vi "INI-FGV2.vi"(6 "Enum":T1, 8 "Raw String? (F)":bool, 9 ">> Section >>":string, 10 ">> Default Value >>":string, 11 ">> Variable Name >>":string) -> (0 "error out":errorcluster, 2 "Key?":bool, 3 "Value":string)   [LabVIEW 2017, in "INI-Static-Variable-Support.lvlib"]
uses:
  INI-Static-Variable-Support.lvlib
  _fgv-oper.ctl
  global-csm-ini-db-change-flag.vi
  LabVIEW-Config/Read Key (String).vi
  LabVIEW-Config/LabVIEW-Config.lvlib
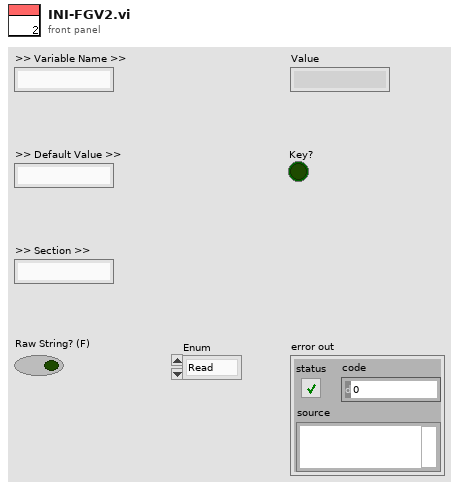
[diagram p1: front panel]
types:
  T1 = typedef "_fgv-oper.ctl" = enum16{"Read", "Write", "Sync"}
  T2 = typedef "LabVIEW-Config.lvlib/Config.ctl" = cluster{"Path":path, "Lines":string[], "Tokens":enum8{"comment", "section", "key"}[], "Modified?":bool}
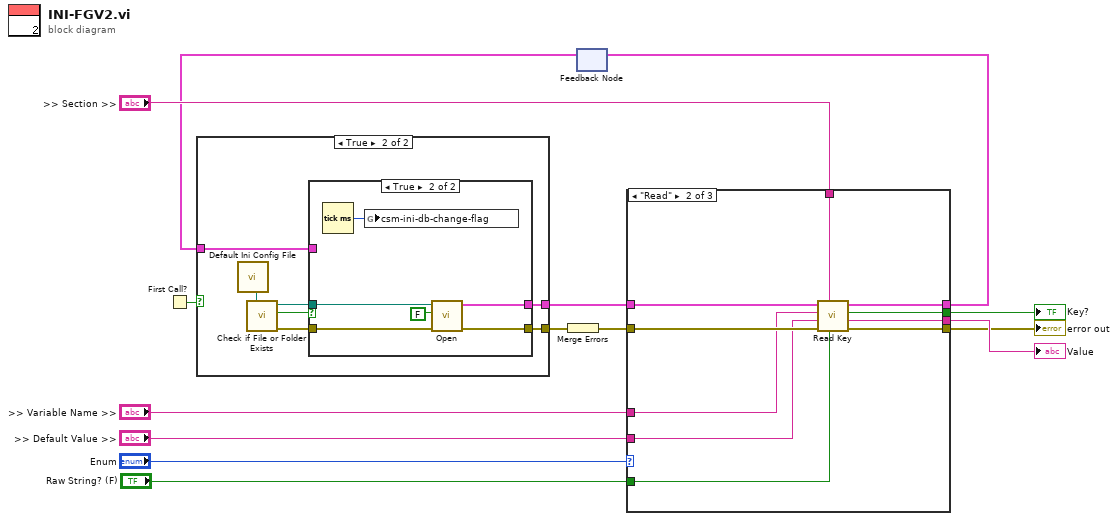
[diagram p0: block diagram]
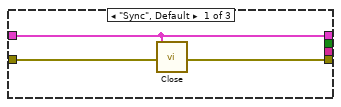
[diagram p2: hidden frame]
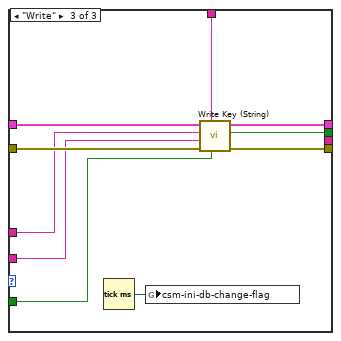
[diagram p3: hidden frame]
diagram:
  n1 = First Call?() -> (First Call?: T/F=w7:bool)
  n2 = feedback #1() -> (w4:T2)  [unwired: 1 in]
  n3 = case shown="True" w7 {
    tunnel: [w15 w19] -> w13
    tunnel: [_ w18] -> w6
    tunnel: w4 -> [w15 w16]
    frame False {
    }
    frame True {
      n4 = call "Default Ini Config File.vi"() -> ("appended path"=w22:path)  [unwired: 11 in]
      n5 = call <vilib>:"Check if File or Folder Exists.vi"("path"=w22) -> ("error out"=w20:errorcluster, "file or folder exists?"=w17:bool, "dup path"=w21:path)  [unwired: 8 in]
      n6 = case shown="True" w17 {
        tunnel: w21 -> [_ w30]
        tunnel: w20 -> [w24 w29]
        tunnel: [w23 w27] -> w19
        tunnel: [w24 w26] -> w18
        tunnel: w16 -> [w23 _]
        frame False {
        }
        frame True {
          n7 = Tick Count (ms)() -> (millisecond timer value=w25:u32)
          n8 = global write "global-csm-ini-db-change-flag.vi" "csm-ini-db-change-flag"(w25) -> ()
          n9 = call "Open.vi"("error in (no error)"=w29, "Create if not exists? (T)"=FALSE, "Path"=w30) -> ("error out"=w26:errorcluster, "Config"=w27:T2)  [unwired: 5 in, 2 out]
        }
      }
    }
  }
  n10 = Merge Errors(w6) -> (w14:errorcluster)
  n11 = case shown="\"Read\"" "Enum" {
    tunnel: w14 -> [w33 w43 w51]
    tunnel: w13 -> [w31 w42 w52]
    tunnel: ">> Section >>" -> [_ w41 w48]
    tunnel: [_ w40 _] -> w11
    tunnel: ">> Default Value >>" -> [_ w39 w47]
    tunnel: ">> Variable Name >>" -> [_ w38 w46]
    tunnel: [w32 w37 w50] -> w8
    tunnel: [w31 w36 w49] -> w5
    tunnel: [_ w35 w45] -> w2
    tunnel: "Raw String? (F)" -> [_ w34 w44]
    frame "Sync", Default {
      n12 = call "Close.vi"("error in (no error)"=w33, "Config"=w31) -> ("error out"=w32:errorcluster)  [unwired: 8 in, 1 out]
    }
    frame "Read" {
      n13 = call-poly "Read Key.vi"("Read Raw String? (F)"=w34, "Section Name"=w41, "error in (no error)"=w43, "Default"=w39, "Key Name"=w38, "Config in"=w42) -> ("error out"=w37:errorcluster, "Value"=w40:string, "Key Found?"=w35:bool, "Config out"=w36:T2)  [unwired: 2 in]
    }
    frame "Write" {
      n14 = Tick Count (ms)() -> (millisecond timer value=w53:u32)
      n15 = global write "global-csm-ini-db-change-flag.vi" "csm-ini-db-change-flag"(w53) -> ()
      n16 = call "Write Key (String).vi"("Write Raw String? (F)"=w44, "Section Name"=w48, "error in (no error)"=w51, "Value"=w47, "Key Name"=w46, "Config in"=w52) -> ("error out"=w50:errorcluster, "Key Replaced?"=w45:bool, "Config out"=w49:T2)  [unwired: 3 in]
    }
  }
  "Value" <- w11
  "error out" <- w8
  "Key?" <- w2
  n17 = feedback-in #1(w5) -> ()
